vi "InstanceNumberCounter.vi"(7 "Action":enum16{"Get", "Add", "Subtract"}(ring), 8 "error in (no error)":errorcluster, 11 "VI Activation in":refnum<class "VIActivation.lvclass">) -> (0 "error out":errorcluster, 2 "InstanceNumber out":i32, 3 "VI Activation out":refnum<class "VIActivation.lvclass">)   [LabVIEW 2021, in "VIActivation.lvlib" / "VIActivation.lvclass"]
uses:
  VIActivation.lvclass
  VIActivation.lvclass/VIActivation.ctl
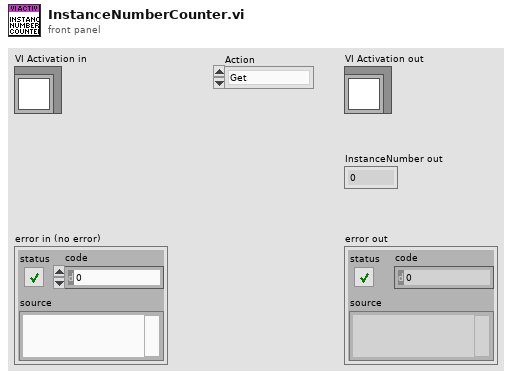
[diagram p1: front panel]
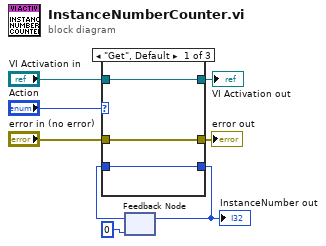
[diagram p0: block diagram]
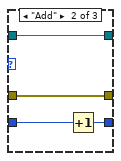
[diagram p2: hidden frame]
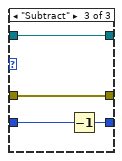
[diagram p3: hidden frame]
diagram:
  n1 = feedback #1(0 ("InstanceNumber out")) -> (w7:i32)
  n2 = case shown="\"Get\", Default" "Action" {
    tunnel: [w10 w14 w18] -> w8
    tunnel: w7 -> [w10 w15 w19]
    tunnel: "error in (no error)" -> [w9 w13 w16]
    tunnel: [w9 w13 w16] -> w3
    tunnel: "VI Activation in" -> [w11 w12 w17]
    tunnel: [w11 w12 w17] -> w1
    frame "Get", Default {
    }
    frame "Add" {
      n3 = Increment(x=w15) -> (x+1=w14:i32)
    }
    frame "Subtract" {
      n4 = Decrement(x=w19) -> (x-1=w18:i32)
    }
  }
  "VI Activation out" <- w1
  "error out" <- w3
  "InstanceNumber out" <- w8
  n5 = feedback-in #1(w8) -> ()
